vi "SetMargin.vi"(0 "handle in":i32, 1 "UnitAddress(0)":u16, 2 "MotNr(0..5)":u8, 5 "error in":errorcluster, 7 "Margin(0)":u16) -> (14 "handle out":i32, 19 "error out":errorcluster)   [LabVIEW 2014, in "Sixpack - Driver.lvlib"]
doc: "Dieser Befehl ermöglicht es, bei linearen Antrieben ein Spiel des Referenzschalters auszugleichen. Es wird bei der Referenzfahrt um Margin weiter in den Referenzschalter hinein gefahren und der Referenzpunkt erst dort gesetzt. Dies ist sinnvoll, wenn die Referenzpunktüberprüfung (siehe SetMotorParameters, MT_TESTNULL) verwendet wird. \n\nCMD $1A\nMotorNr (0...5)\nMargin (0..65535)"
uses:
  Sixpack - Driver.lvlib
  DLL/PackDLL.dll
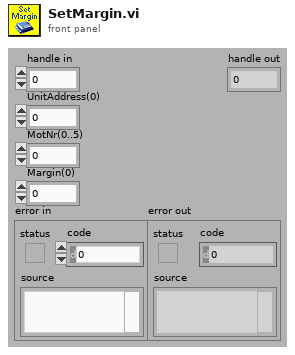
[diagram p1: front panel]
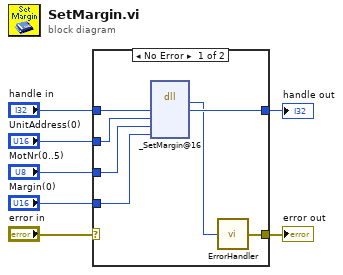
[diagram p0: block diagram]
diagram:
  n1 = case shown="No Error" "error in" {
    selector: "error in" -> [_ w15]
    tunnel: "handle in" -> [w14 w16]
    tunnel: [w13 w16] -> w6
    tunnel: "UnitAddress(0)" -> [w12 _]
    tunnel: "MotNr(0..5)" -> [w11 _]
    tunnel: "Margin(0)" -> [w10 _]
    tunnel: [w8 w15] -> w2
    frame No Error {
      n2 = dll-call lib="D:/CS-Source/LV2014/GPL/instr.lib/SixPack/PackDLL/DLL/PackDLL.dll" fn="_SetMargin@16" label="SetMargin"("HANDLE"=w14, "UnitAddress"=w12, "MotNr"=w11, "Margin"=w10) -> ("BOOLEAN"=w9:i8, "HANDLE"=w13:i32)  [unwired: 6 in, 2 out]
      n3 = call "ErrorHandler.vi"("BOOLEAN"=w9) -> ("error out"=w8:errorcluster)
    }
    frame Error {
    }
  }
  "handle out" <- w6
  "error out" <- w2
